vi "Get Generic Devices.vi"(11 "Supported Device Code":u32[](array[numeric])) -> (3 "Supported Device Full Name":string[](array[string]))   [LabVIEW 2021, in "myRIOMetaDataObj.lvclass"]
uses:
  myRIOMetaDataObj.lvclass
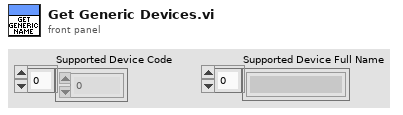
[diagram p1: front panel]
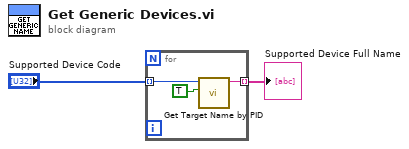
[diagram p0: block diagram]
diagram:
  n1 = for {
    tunnel: "Supported Device Code" -> [w5] mode=indexing
    tunnel: [w3] -> w1 mode=indexing
    n2 = call <vilib>:"Get Target Name by PID.vi"("Full Name?"=TRUE, "Device Model"=w5) -> ("Device Model Str"=w3:string)  [unwired: 8 in, 1 out]
  }
  "Supported Device Full Name" <- w1
